vi "Friction.vi"   [LabVIEW 2017, in "NI_AdvCtrl_nonlinear.lvlib"]
doc: "LabVIEW no longer supports this VI. You can obtain similar functionality by installing the LabVIEW Simulation Module.\n\nRealizes a discontinuity at zero but guarantees the linear behavior elsewhere."
uses:
  <vilib>/addons/control/advanced/NI_AdvCtrl_nonlinear.lvlib
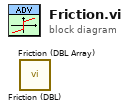
[diagram p0: block diagram]
diagram:
  n1 = call <vilib>:"Friction (DBL).vi"() -> ()  [unwired: 4 in, 1 out]
  n2 = call <vilib>:"Friction (DBL Array).vi"() -> ()  [unwired: 4 in, 1 out]
